vi "MRC Alert Set Alert Text.vi"(8 "error in (no error)":errorcluster, 10 "text":T1, 11 "handle":i64) -> (0 "error out":errorcluster)   [LabVIEW 2026, in "MrcLib.lvlib"]
doc: "MRC_Status MRC_CALLCONV MRC_Alert_SetAlertText(MRC_AlertHandle handle,\n const struct MRC_String* text);"
uses:
  MrcLib.lvlib
  MrcLib.dll
  <vilib>/MRC/Types/MRC String.ctl
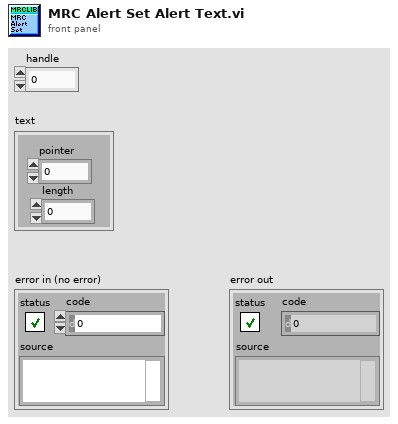
[diagram p1: front panel]
types:
  T1 = typedef "MRC String.ctl" = cluster{"pointer":u64, "length":u64}
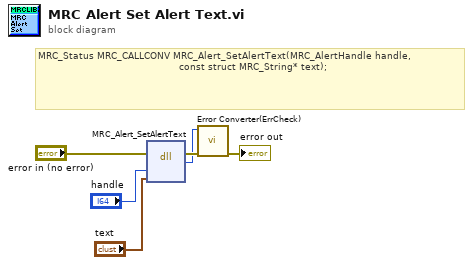
[diagram p0: block diagram]
diagram:
  # "MRC_Status MRC_CALLCONV MRC_Alert_SetAlertText(MRC_AlertHandle handle,\n                                               const struct MRC_String* text);"
  n1 = dll-call lib="MrcLib.*" fn="MRC_Alert_SetAlertText"(error in="error in (no error)", "handle"="handle", "text"="text") -> (error out=w2:errorcluster, w1:i32)  [unwired: 4 in, 1 out]
  n2 = call <vilib>:"Error Converter(ErrCheck).vi"("error in (no error)"=w2, "status"=w1) -> ("error out"=→"error out":errorcluster)  [unwired: 9 in]
